vi "Get FP size.vi"(8 "error in (no error)":errorcluster, 11 "VI Refnum":refnum<vi>) -> (0 "error out":errorcluster, 1 "Height":i16, 2 "Width":i16, 3 "VI Refnum out":refnum<vi>)   [LabVIEW 2014, in "COSYLib.lvlib"]
uses:
  COSYLib.lvlib
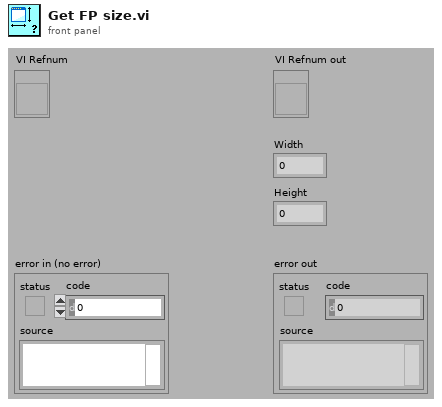
[diagram p1: front panel]
types:
  T1 = typedef "LVRectTypeDef.ctl" = cluster{"Left":i16, "Top":i16, "Right":i16, "Bottom":i16}
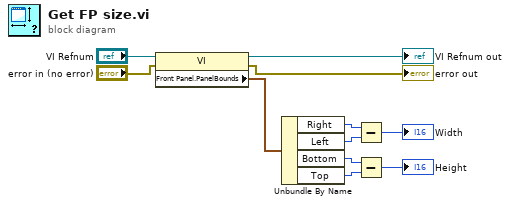
[diagram p0: block diagram]
diagram:
  n1 = property class="VI"(reference="VI Refnum", error in="error in (no error)") -> (reference out=→"VI Refnum out":refnum<vi>, error out=→"error out":errorcluster, "Front Panel.PanelBounds"=w10:T1)
  n2 = Unbundle By Name(w10) -> ("Right"=w6:i16, "Left"=w5:i16, "Bottom"=w4:i16, "Top"=w3:i16)
  n3 = Subtract(x=w6, y=w5) -> (x-y=→"Width":i16)
  n4 = Subtract(x=w4, y=w3) -> (x-y=→"Height":i16)
